vi "programacion 6 Lester Roche.vi"() -> ()   [LabVIEW 2011]
panel:
  out "Alarma":bool
  out "Temperatura":i32(slide) scale=0.0..100.0
  out "Cuarta":bool
  out "Tercera":bool
  out "Segunda":bool
  out "Primera":bool
  out "Velocidad":i32(knob) scale=0.0..180.0
  # "Debera de generar la velocidad en numero entero. \nLuego de acuerdo a la siguiente tabla:\n1-30 primera\n31-50 segunda\n51-85 tercera \n86-180 cuarta\ndebera de encender las luces de los cambios.\nEncender la alarma cuando la temperatura sobrepase \nlos 80 grados y la velocidad es mayor a 150."
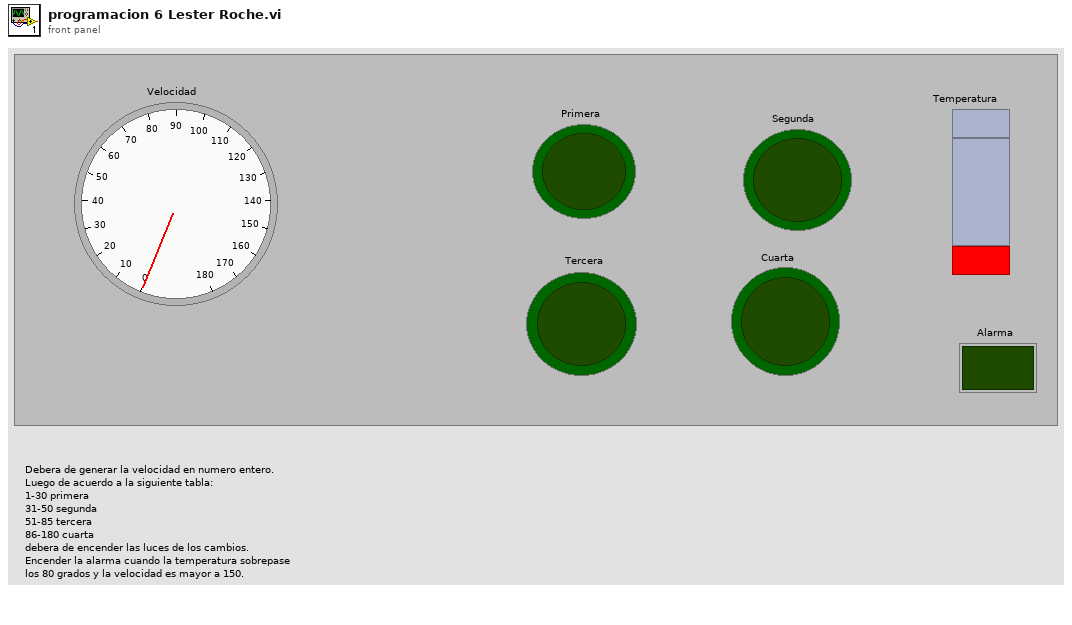
[diagram p1: front panel]
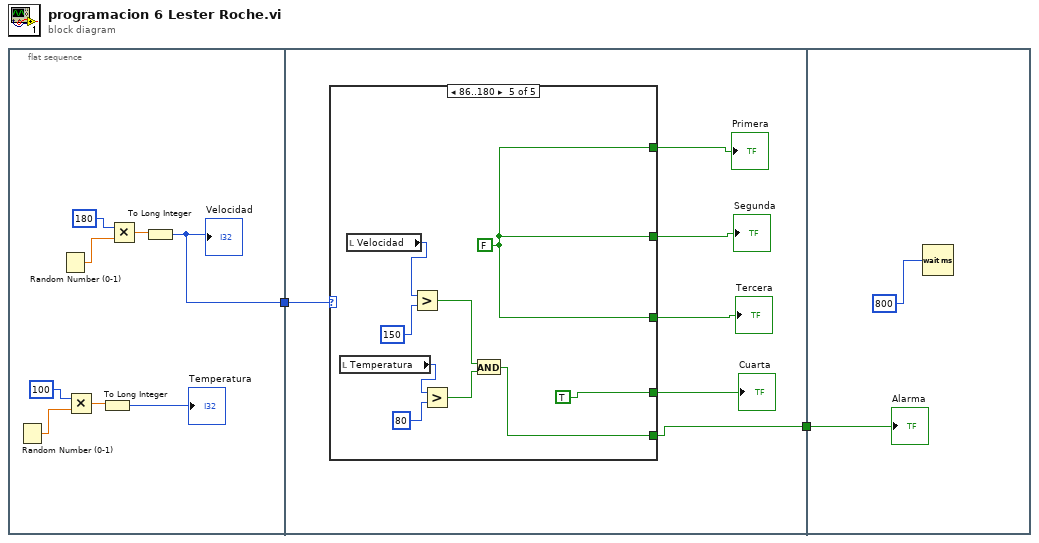
[diagram p0: block diagram]
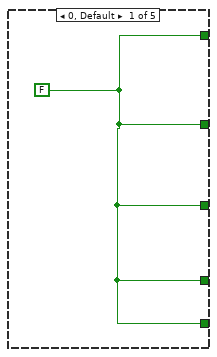
[diagram p2: hidden frame]
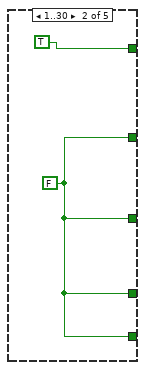
[diagram p3: hidden frame]
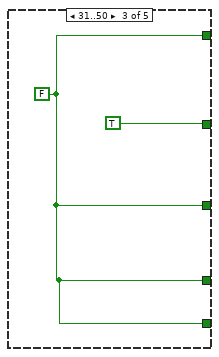
[diagram p4: hidden frame]
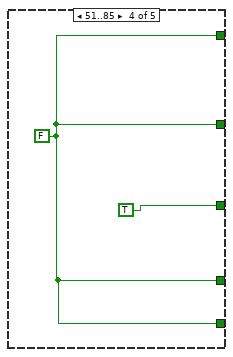
[diagram p5: hidden frame]
diagram:
  n1 = flat-sequence {
    tunnel: [w7] -> w2
    tunnel: w2 -> [w16]
    tunnel: [w11] -> w1
    tunnel: w1 -> [w33]
    frame #0 {
      n2 = Random Number (0-1)() -> (number: 0 to 1=w6:dbl)
      n3 = Random Number (0-1)() -> (number: 0 to 1=w8:dbl)
      n4 = Multiply(x=100, y=w6) -> (x*y=w4:dbl)
      n5 = To Long Integer(number=w4) -> (32bit integer=→"Temperatura":i32)
      n6 = Multiply(x=180, y=w8) -> (x*y=w10:dbl)
      n7 = To Long Integer(number=w10) -> (32bit integer=w7:i32)
      "Velocidad" <- w7
    }
    frame #1 {
      n8 = case shown="86..180" w16 {
        tunnel: [w17 TRUE w20 w22 w31] -> w15
        tunnel: [w17 w18 TRUE w22 w31] -> w14
        tunnel: [w17 w18 w20 TRUE w31] -> w13
        tunnel: [w17 w18 w20 w22 TRUE] -> w12
        tunnel: [w17 w18 w20 w22 w24] -> w11
        frame 0, Default {
          w17 = FALSE
        }
        frame 1..30 {
          w18 = FALSE
        }
        frame 31..50 {
          w20 = FALSE
        }
        frame 51..85 {
          w22 = FALSE
        }
        frame 86..180 {
          w31 = FALSE
          n9 = local read "Temperatura"() -> (w27:i32)
          n10 = local read "Velocidad"() -> (w29:i32)
          n11 = Greater?(x=w29, y=150) -> (0:w26:bool)
          n12 = Greater?(x=w27, y=80) -> (0:w25:bool)
          n13 = And(x=w26, y=w25) -> (x .and. y?=w24:bool)
        }
      }
      "Primera" <- w15
      "Segunda" <- w14
      "Tercera" <- w13
      "Cuarta" <- w12
    }
    frame #2 {
      n14 = Wait (ms)(milliseconds to wait=800) -> ()  [unwired: 1 out]
      "Alarma" <- w33
    }
  }
